vi "Write _ServiceName.vi"(8 "error in (no error)":errorcluster, 10 "_ServiceName":string, 11 "Session in":refnum<class "Session.lvclass">) -> (0 "error out":errorcluster, 3 "Session out":refnum<class "Session.lvclass">)   [LabVIEW 2015, in "NI_Azure_Core.lvlib" / "Session.lvclass"]
uses:
  Session.lvclass
  Session.lvclass/Session.ctl
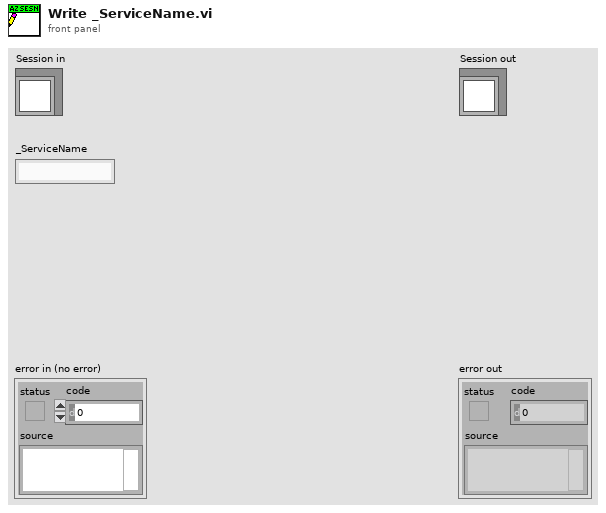
[diagram p1: front panel]
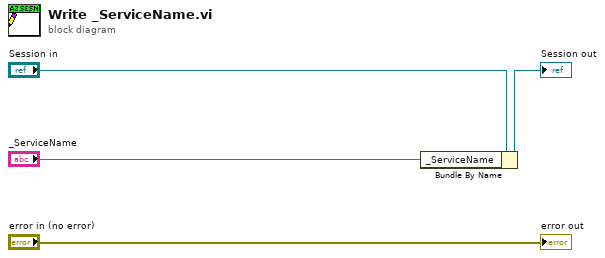
[diagram p0: block diagram]
diagram:
  n1 = Bundle By Name(cluster="Session in", "_ServiceName"="_ServiceName") -> (→"Session out":refnum<class "Session.lvclass">)
  "error out" <- "error in (no error)"
